vi "String to WSTRING Byte Stream.vi"(8 "error in (no error)":errorcluster, 10 "Value":string) -> (0 "error out":errorcluster, 2 "Byte Stream":u8[](array[numeric]))   [LabVIEW 2018, in "TwinCAT ADS.lvclass"]
uses:
  TwinCAT ADS.lvclass
  TwinCAT.Ads
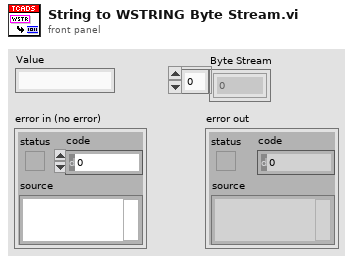
[diagram p1: front panel]
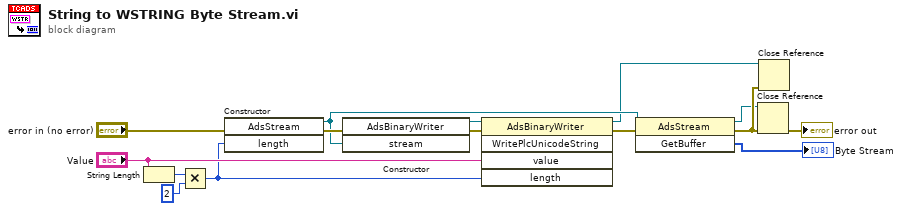
[diagram p0: block diagram]
diagram:
  n1 = String Length(string="Value") -> (length=w1:i32)
  n2 = Multiply(x=w1, y=2) -> (x*y=w2:i32)
  n3 = constructor class="AdsStream"(error in="error in (no error)", "length"=w2) -> (reference out=w11:refnum<k24>, error out=w13:errorcluster)  [unwired: 2 in, 2 out]
  n4 = constructor class="AdsBinaryWriter"(error in=w13, "stream"=w11) -> (reference out=w15:refnum<k24>, error out=w14:errorcluster)  [unwired: 2 in, 2 out]
  n5 = invoke class="AdsBinaryWriter" method="WritePlcUnicodeString"(reference=w15, error in=w14, "value"="Value", "length"=w2) -> (reference out=w7:refnum<k24>, error out=w12:errorcluster)  [unwired: 1 in, 3 out]
  n6 = invoke class="AdsStream" method="GetBuffer"(reference=w11, error in=w12) -> (reference out=w8:refnum<k24>, error out=w9:errorcluster, "GetBuffer"=→"Byte Stream":u8[])  [unwired: 1 in]
  n7 = Close Reference(reference=w8, error in (no error)=w9) -> (error out=→"error out":errorcluster)
  n8 = Close Reference(reference=w7, error in (no error)=w9) -> ()  [unwired: 1 out]
